vi "WPI_CameraDirectly from IP Camera.vi"(5 "port":u16=80, 7 "Operation":enum16{"Read", "Reopen", "Close"}(ring), 8 "error in":errorcluster, 9 "Camera Settings":T3={"name"="", "fps"=30, "compression"=30, "Image Size"=enum."320x240"}, 10 "Image":T1, 11 "address":string="10.te.am.11") -> (0 "error out":errorcluster, 1 "Bandwidth (Mbps)":dbl=30.0, 2 "Image Out":T1)   [LabVIEW 2017]
doc: "This VI is intended for testing, examples, and demos. It assumes the camera is directly accssible from the computer and not the robot. It retrieves an image from either a USB or IP Axis camera.\n\nThis software is licensed. Open the labview\\readme\\WPI Robotics Library Open Source License.txt file for more information."
uses:
  <vilib>/Rock Robotics/WPI/Camera/WPI_CameraImageSize.ctl
  <vilib>/vision/Image Controls.llb/IMAQ Image.ctl
  <vilib>/picture/picture.llb/imagedata.ctl
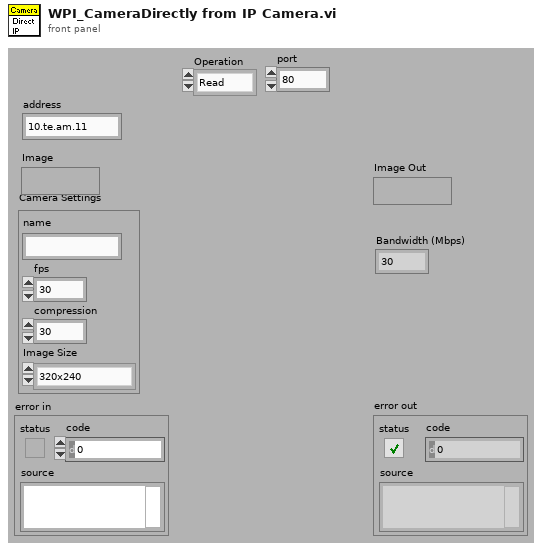
[diagram p1: front panel]
types:
  T1 = typedef "IMAQ Image.ctl" = refnum<image>
  T2 = typedef "WPI_CameraImageSize.ctl" = enum16{"640x480", "320x240", "160x120", "Custom"}
  T3 = cluster{"name":string, "fps":i32, "compression":i32, "Image Size":T2}
  T4 = typedef "imagedata.ctl" = cluster{"image type":i32, "image depth":i32, "image":u8[], "mask":u8[], "colors":u32[], "Rectangle":cluster{"left":i16, "top":i16, "right":i16, "bottom":i16}}
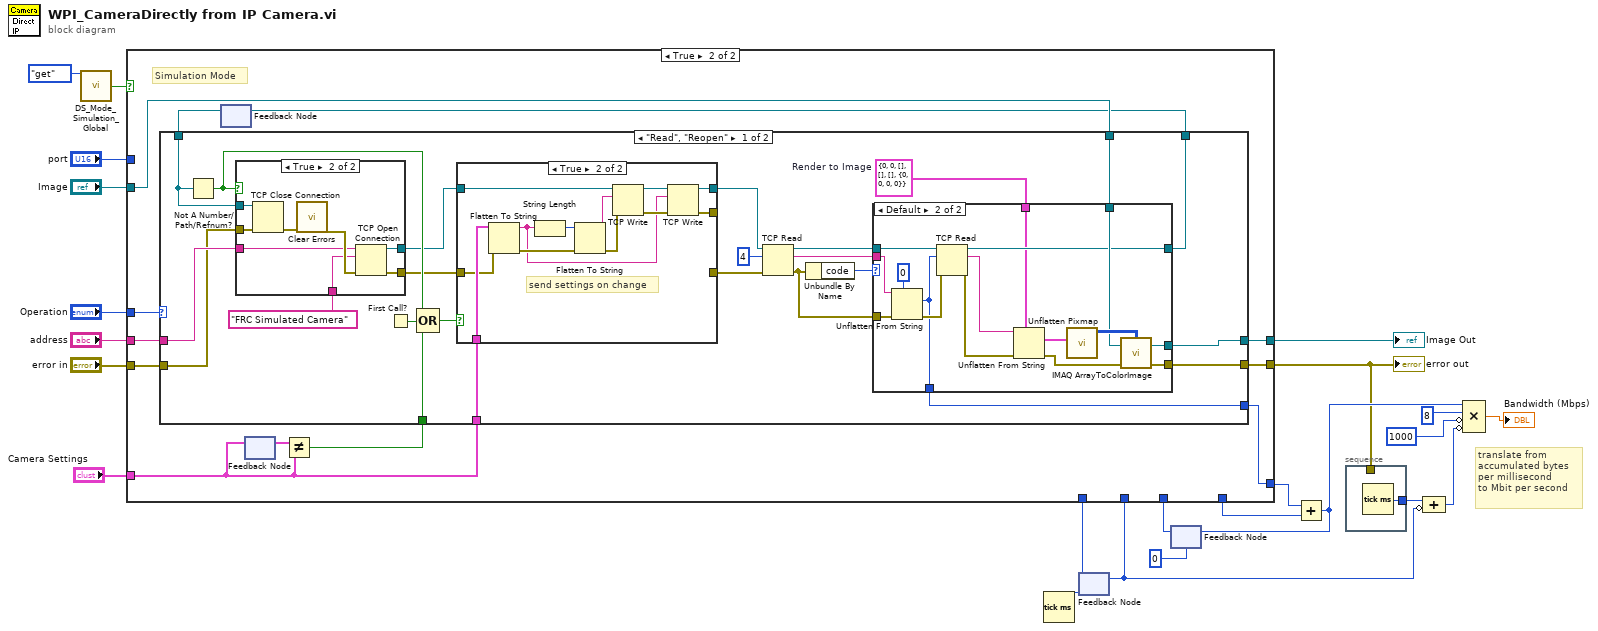
[diagram p0: block diagram]
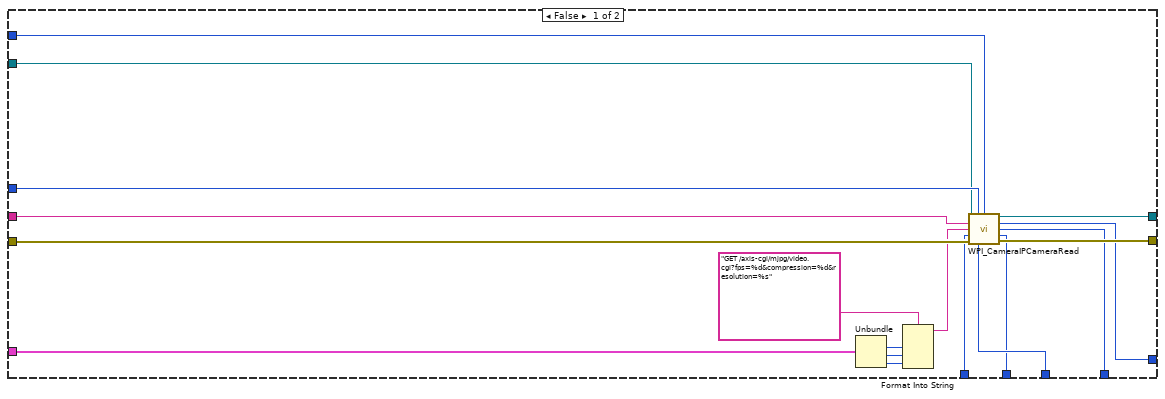
[diagram p2: hidden frame]
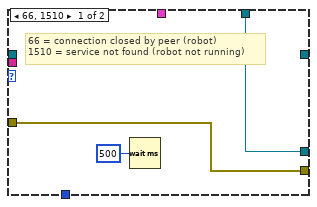
[diagram p4: hidden frame]
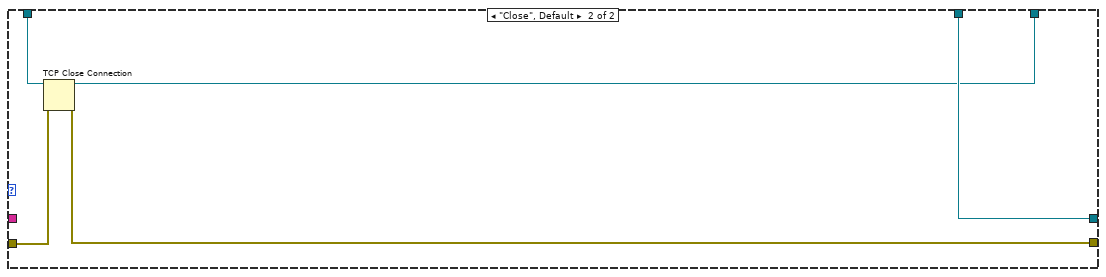
[diagram p6: hidden frame]
diagram:
  # "translate from\naccumulated bytes\nper millisecond \nto Mbit per second"
  n1 = call <vilib>:"DS_Mode_Simulation_Global.vi"("menu"=enum16{"set", "get"}."get") -> ("simulated? out"=w18:bool)  [unwired: 13 in, 1 out]
  n2 = Tick Count (ms)() -> (millisecond timer value=w15:u32)
  n3 = feedback #1(w15) -> (w10:u32)
  n4 = feedback #2(0) -> (w12:i32)
  n5 = case shown="True" w18 {
    tunnel: "error in" -> [w41 w52]
    tunnel: "address" -> [w31 w53]
    tunnel: [w40 w51] -> w21
    tunnel: [w39 w50] -> w5
    tunnel: "Operation" -> [w38 w48]
    tunnel: "Image" -> [w37 w49]
    tunnel: [w36 w43] -> w8
    tunnel: w12 -> [w35 _]
    tunnel: [w34 _] -> w11
    tunnel: w10 -> [w33 _]
    tunnel: [w32 _] -> w6
    tunnel: "Camera Settings" -> [w30 w45]
    tunnel: "port" -> [w29 _]
    frame False {
      n6 = Unbundle(w30) -> ("fps"=w28:i32, "compression"=w27:i32, "Image Size"=w26:T2)  [unwired: 1 out]
      n7 = Format Into String(format string="GET /axis-cgi/mjpg/video.cgi?fps=%d&compression=%d&resolution=%s", w28, w27, w26) -> (resulting string=w24:string)  [unwired: 2 in, 1 out]
      n8 = call <vilib>:"WPI_CameraIPCameraRead.vi"("Refnum in"=w37, "Operation"=w38, "port"=w29, "address"=w31, "cgi string"=w24, "millisecs in"=w33, "error in (no error)"=w41, "accum length in"=w35) -> ("Refnum out"=w40:T1, "length"=w36:i32, "accum length out"=w34:i32, "millisecs out"=w32:u32, "error out"=w39:errorcluster)  [unwired: 3 in]
    }
    frame True {
      # "Simulation Mode"
      n9 = feedback #3() -> (w42:refnum<k5>)  [unwired: 1 out]
      n10 = feedback-in #4(w45) -> ()
      n11 = feedback #4() -> (w46:T3)  [unwired: 1 in]
      n12 = Not Equal?(x=w46, y=w45) -> (x != y?=w44:bool)
      n13 = case shown="\"Read\", \"Reopen\"" w48 {
        tunnel: w53 -> [w77 _]
        tunnel: w52 -> [w76 w125]
        tunnel: [w75 w123] -> w51
        tunnel: [w67 w124] -> w50
        tunnel: w49 -> [w74 w123]
        tunnel: [w69 _] -> w43
        tunnel: w45 -> [w60 _]
        tunnel: [w68 w122] -> w47
        tunnel: w44 -> [w64 _]
        tunnel: w42 -> [w55 w121]
        frame "Read", "Reopen" {
          w54 = T4 {"image type"=0, "image depth"=0, "image"=[], "mask"=[], "colors"=[], "Rectangle"={"left"=0, "top"=0, "right"=0, "bottom"=0}}  # Render to Image
          n14 = Not A Number/Path/Refnum?(number/path/refnum=w55) -> (NaN/Path/Refnum?=w63:bool)
          n15 = case shown="True" w63 {
            tunnel: w55 -> [w112 w120]
            tunnel: w77 -> [_ w114]
            tunnel: [w112 w117] -> w62
            tunnel: w76 -> [w111 w116]
            tunnel: [w111 w115] -> w59
            tunnel: "FRC Simulated Camera" ("service name") -> [_ w113]
            frame False {
            }
            frame True {
              n16 = TCP Close Connection(connection ID=w120, error in (no error)=w116) -> (error out=w119:errorcluster)  [unwired: 2 out]
              n17 = call <vilib>:"Clear Errors.vi"("error in (no error)"=w119) -> ("error out"=w118:errorcluster)  [unwired: 1 in, 5 out]
              n18 = TCP Open Connection(address=w114, remote port or service name=w113, error in (no error)=w118) -> (connection ID=w117:refnum<k5>, error out=w115:errorcluster)  [unwired: 2 in]
            }
          }
          n19 = First Call?() -> (First Call?: T/F=w66:bool)
          n20 = Compound Arithmetic op=OR(w63, w66, w64) -> (w65:bool)
          n21 = case shown="True" w65 {
            tunnel: w62 -> [w79 w91]
            tunnel: w60 -> [_ w89]
            tunnel: [w79 w82] -> w61
            tunnel: w59 -> [w78 w81]
            tunnel: [w78 _] -> w58
            tunnel: [_ w80] -> _
            frame False {
            }
            frame True {
              # "send settings on change"
              n22 = Flatten To String(anything=w89, error in (no error)=w81) -> (data string=w83:string, error out=w85:errorcluster)  [unwired: 2 in, 1 out]
              n23 = String Length(string=w83) -> (length=w90:i32)
              n24 = Flatten To String(anything=w90, error in (no error)=w85) -> (data string=w88:string, error out=w86:errorcluster)  [unwired: 2 in, 1 out]
              n25 = TCP Write(connection ID=w91, data in=w88, error in (no error)=w86) -> (connection ID out=w84:refnum<k5>, error out=w87:errorcluster)  [unwired: 1 in, 1 out]
              n26 = TCP Write(connection ID=w84, data in=w83, error in (no error)=w87) -> (connection ID out=w82:refnum<k5>, error out=w80:errorcluster)  [unwired: 1 in, 1 out]
            }
          }
          n27 = TCP Read(connection ID=w61, bytes to read=4, error in (no error)=w58) -> (connection ID out=w71:refnum<k5>, data out=w72:string, error out=w56:errorcluster)  [unwired: 1 in, 1 out]
          n28 = Unbundle By Name(w56) -> ("code"=w70:i32)
          n29 = case shown="Default" w70 {
            tunnel: [w94 w107] -> w75
            tunnel: [w93 w96] -> w67
            tunnel: w74 -> [w94 w106]
            tunnel: w72 -> [_ w105]
            tunnel: w71 -> [_ w104]
            tunnel: w56 -> [w93 w102]
            tunnel: [_ w100] -> w69
            tunnel: [_ w97] -> w68
            tunnel: w54 -> [_ w95]
            frame 66, 1510 {
              # "66 = connection closed by peer (robot)\n1510 = service not found (robot not running)"
              n30 = Wait (ms)(milliseconds to wait=u32 500) -> ()  [unwired: 1 out]
            }
            frame Default {
              n31 = Unflatten From String(type=0 ("bytes to read"), binary string=w105, error in (no error)=w102) -> (value=w100:i32, error out=w101:errorcluster)  [unwired: 2 in, 1 out]
              n32 = TCP Read(connection ID=w104, bytes to read=w100, error in (no error)=w101) -> (connection ID out=w97:refnum<k5>, data out=w108:string, error out=w99:errorcluster)  [unwired: 1 in, 1 out]
              n33 = Unflatten From String(type=w95, binary string=w108, error in (no error)=w99) -> (value=w109:T4, error out=w98:errorcluster)  [unwired: 2 in, 1 out]
              n34 = call <vilib>:"Unflatten Pixmap.vi"("image data"=w109) -> ("24-bit pixmap"=w110:u32[][])  [unwired: 4 in, 6 out]
              n35 = call "IMAQ ArrayToColorImage"("Image Pixels (U32)"=w110, "Image"=w106, "error in (no error)"=w98) -> ("Image Out"=w107:T1, "error out"=w96:errorcluster)  [unwired: 2 in]
            }
          }
        }
        frame "Close", Default {
          n36 = TCP Close Connection(connection ID=w121, error in (no error)=w125) -> (connection ID out=w122:refnum<k5>, error out=w124:errorcluster)  [unwired: 1 out]
        }
      }
      n37 = feedback-in #3(w47) -> ()
    }
  }
  "Image Out" <- w21
  "error out" <- w5
  n38 = feedback-in #1(w6) -> ()
  n39 = Add(x=w8, y=w11) -> (x+y=w9:i32)
  n40 = feedback-in #2(w9) -> ()
  n41 = stacked-sequence {
    tunnel: [w126] -> w7
    tunnel: w5 -> [_]
    frame #0 {
      n42 = Tick Count (ms)() -> (millisecond timer value=w126:u32)
    }
  }
  n43 = Compound Arithmetic op=ADD(w7, invert w6) -> (w4:u32)
  n44 = Compound Arithmetic op=MULTIPLY(w9, 8 ("timeout ms (25000)"), invert 1000 ("timeout ms (25000)"), invert w4) -> (→"Bandwidth (Mbps)":dbl)
